vi "repeat cycle_normal.vi"(8 "error in (no error)":errorcluster caption="에러 입력(에러 없음)", 10 "waveform in":waveform(dbl), 11 "Waveform Obj 입력":refnum<class "Waveform Gen.lvclass">) -> (0 "error out":errorcluster caption="에러 출력", 2 "waveform out":waveform(dbl), 3 "Waveform Obj 출력":refnum<class "Waveform Gen.lvclass">)   [LabVIEW 2020, in "Waveform Gen.lvclass"]
uses:
  Waveform Gen.lvclass
  Waveform Gen.lvclass/Waveform Gen.ctl
  Accessors/Read cycle.vi
  <vilib>/Waveform/WDTOps.llb/WDT Append Waveforms DBL.vi
  <vilib>/Waveform/WDTOps.llb/WDT Number of Waveform Samples DBL.vi
  <vilib>/Waveform/WDTOps.llb/WDT Get Waveform Subset DBL.vi
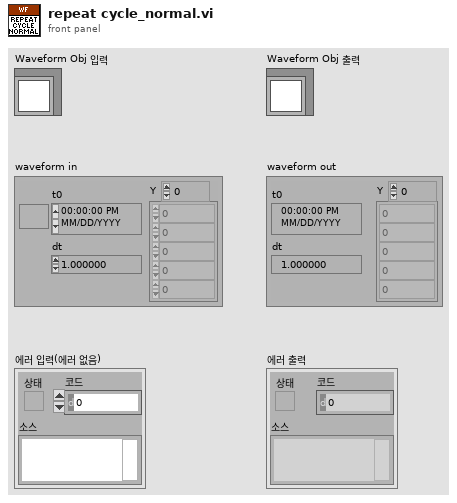
[diagram p1: front panel]
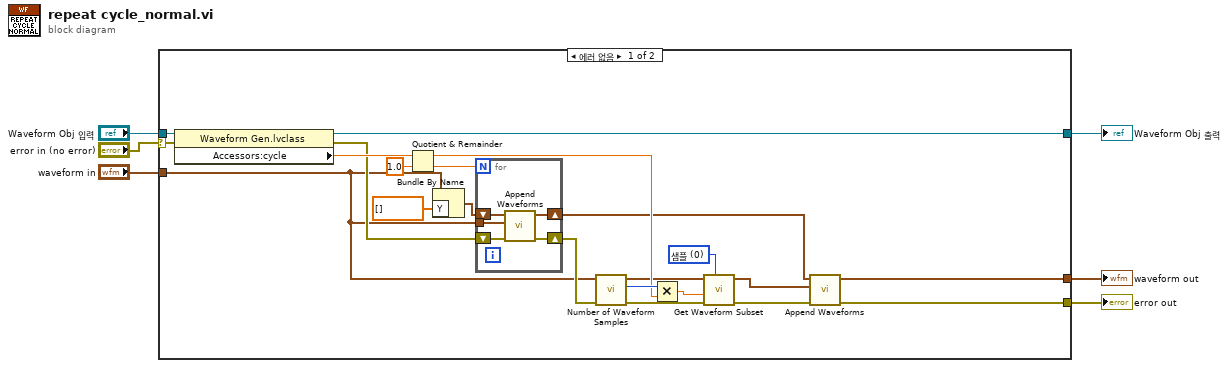
[diagram p0: block diagram]
diagram:
  n1 = case shown="에러 없음" "error in (no error)" {
    selector: "error in (no error)" -> [w25 w35]
    tunnel: [w8 w35] -> w3
    tunnel: "Waveform Obj 입력" -> [w28 w34]
    tunnel: [w9 w34] -> w4
    tunnel: "waveform in" -> [w10 _]
    tunnel: [w7 _] -> w1
    frame No Error {
      w15 = u16 0 items=["샘플", "상대 시간"] ("start/duration format")
      n2 = property class="Waveform Gen.lvclass"(reference=w28, error in=w25) -> (reference out=w9:refnum<class "Waveform Gen.lvclass">, error out=w19:errorcluster, "Accessors:cycle"=w27:dbl)
      n3 = Quotient & Remainder(x=w27, y=1.0) -> (x-y*floor(x/y)=w22:dbl, floor(x/y)=w24:dbl)
      n4 = Bundle By Name(cluster=w10, "Y"=dbl[] []) -> (w12:waveform(dbl))
      n5 = for {
        N: w24 -> [_]
        shift-right: [w32] -> w11
        shift-left: w12 -> [w33]
        shift-right: [w30] -> w18
        shift-left: w19 -> [w31]
        tunnel: w10 -> [w29]
        n6 = call-poly <vilib>:"Append Waveforms.vi"("error in (no error)"=w31, "waveform B"=w29, "waveform A"=w33) -> ("error out"=w30:errorcluster, "waveform out"=w32:waveform(dbl))  [unwired: 7 in]
      }
      n7 = call-poly <vilib>:"Number of Waveform Samples.vi"("error in (no error)"=w18, "waveform in"=w10) -> ("error out"=w20:errorcluster, "number of samples"=w23:i32, "waveform out"=w16:waveform(dbl))  [unwired: 7 in]
      n8 = Multiply(x=w23, y=w22) -> (x*y=w21:dbl)
      n9 = call-poly <vilib>:"Get Waveform Subset.vi"("start/duration format"=w15, "error in (no error)"=w20, "duration"=w21, "waveform in"=w16) -> ("error out"=w17:errorcluster, "waveform out"=w14:waveform(dbl))  [unwired: 2 in, 2 out]
      n10 = call-poly <vilib>:"Append Waveforms.vi"("error in (no error)"=w17, "waveform B"=w14, "waveform A"=w11) -> ("error out"=w8:errorcluster, "waveform out"=w7:waveform(dbl))  [unwired: 7 in]
    }
    frame Error {
    }
  }
  "error out" <- w3
  "Waveform Obj 출력" <- w4
  "waveform out" <- w1
